vi "PI Convert 1.0 - 1.2 to 1.3.vi"(1 "Prompted Inputs 1.0 - 1.2 Test Parameters":T2={"Tag"="", "Use Instrument"=FALSE, "Quick Mode"=FALSE, "Blank Screen"=FALSE, "Limits"=[], "Reports"={"Reports to Generate"=[], "Print Reports"=TRUE}, "Prompted Items"=[]}) -> (0 "Prompted Inputs 1.3 Test Parameters":T1={"Tag"="", "Use Instrument"=FALSE, "Quick Mode"=FALSE, "Blank Screen"=FALSE, "Limits"=[], "Datasheets"={"Datasheets to Generate"=[], "Print Datasheets"=TRUE}, "Prompted Items"=[]})   [LabVIEW 2011]
uses:
  TypeDefs/PI Test Parameters v1.0-1.2.ctl
  TypeDefs/PI Test Parameters v1.3.ctl
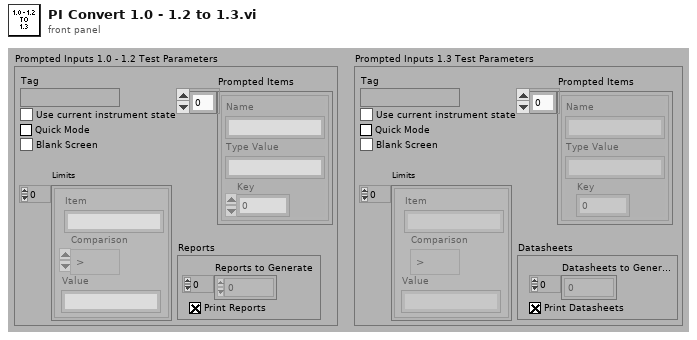
[diagram p1: front panel]
types:
  T1 = typedef "PI Test Parameters v1.3.ctl" = cluster{"Tag":string, "Use Instrument":bool, "Quick Mode":bool, "Blank Screen":bool, "Limits":cluster{"Item":string, "Comparison":enum16{">", ">=", "<", "<=", "<>", "="}, "Value":string}[], "Datasheets":cluster{"Datasheets to Generate":i32[], "Print Datasheets":bool}, "Prompted Items":cluster{"Name":string, "Type Value":string, "Key":i32}[]}
  T2 = typedef "PI Test Parameters v1.0-1.2.ctl" = cluster{"Tag":string, "Use Instrument":bool, "Quick Mode":bool, "Blank Screen":bool, "Limits":cluster{"Item":string, "Comparison":enum16{">", ">=", "<", "<="}, "Value":string}[], "Reports":cluster{"Reports to Generate":i32[], "Print Reports":bool}, "Prompted Items":cluster{"Name":string, "Type Value":string, "Key":i32}[]}
  T3 = cluster{"Item":string, "Comparison":enum16{">", ">=", "<", "<="}, "Value":string}[]
  T4 = cluster{"Reports to Generate":i32[], "Print Reports":bool}
  T5 = cluster{"Name":string, "Type Value":string, "Key":i32}[]
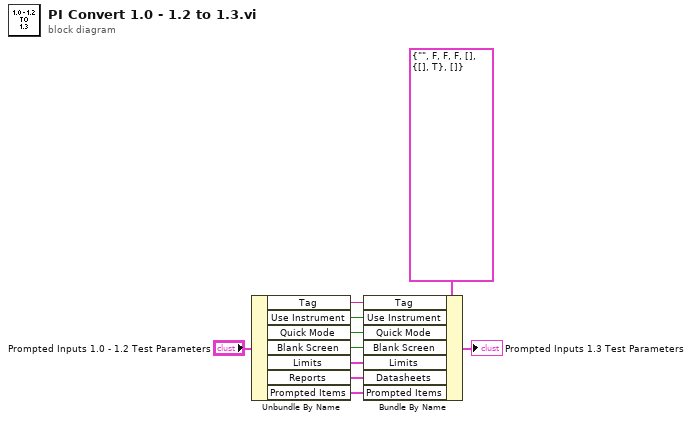
[diagram p0: block diagram]
diagram:
  n1 = Unbundle By Name("Prompted Inputs 1.0 - 1.2 Test Parameters") -> ("Tag"=w4:string, "Use Instrument"=w5:bool, "Quick Mode"=w6:bool, "Blank Screen"=w7:bool, "Limits"=w8:T3, "Reports"=w9:T4, "Prompted Items"=w10:T5)
  n2 = Bundle By Name(cluster=T1 {"Tag"="", "Use Instrument"=FALSE, "Quick Mode"=FALSE, "Blank Screen"=FALSE, "Limits"=[], "Datasheets"={"Datasheets to Generate"=[], "Print Datasheets"=TRUE}, "Prompted Items"=[]} ("Prompted Inputs Test Parameters"), "Tag"=w4, "Use Instrument"=w5, "Quick Mode"=w6, "Blank Screen"=w7, "Limits"=w8, "Datasheets"=w9, "Prompted Items"=w10) -> (→"Prompted Inputs 1.3 Test Parameters":T1)
